vi "Deployment on cDAQ.vi"() -> ()   [LabVIEW 2018]
uses:
  <vilib>/Utility/error.llb/DialogType.ctl
  <vilib>/addons/AML/Data/Common/Controls/aml_Load Data Mode.ctl
  <vilib>/DAQmx/read.llb/DAQmx Read (Analog 2D DBL NChan NSamp).vi
  <vilib>/DAQmx/create/channels.llb/DAQmx Create Channel (AI-Voltage-Basic).vi
  <vilib>/DAQmx/configure/timing.llb/DAQmx Timing (Sample Clock).vi
  <vilib>/DAQmx/miscellaneous.llb/DAQmx Fill In Error Info.vi
  <vilib>/addons/AML/Data/Load Testing Data (2D Array).vi
  <vilib>/addons/AML/Analytics and Machine Learning.lvlib
panel:
  out "Fan status":bool
  out "Predicted probability":dbl[][](array[numeric])=[[0.8062356533229831, 0.19376434667701692]]
  out "Fan status":string="Fan work normal"
  in  "Model file (JSON)":path
  out "Waveform Graph":dbl[][](graph)=[[2.468674629981, 2.468664258944, 2.4700015126559998, 2.469919154421, 2.4675917717059996, 2.4693054330549997, 2.4665564981889996, 2.468985761091, 2.4669664591809997, 2.4659696195069998, 2.466726705208, 2.468710013519, 2.4686398565039998, 2.4688588684029997, 2.468429385459, 2.4684312156419996, 2.467338596391, 2.4671134838819997, 2.4691803705499997, 2.4681774302659996, 2.4676314256709997, 2.46913766628, 2.4677333058579998, 2.467753437871, 2.467754047932, 2.469128515365, 2.4683372662479997, 2.4666229948379996, 2.4670555280869997, 2.466956088144, 2.4668102835649997, 2.46747219975, 2.467281860718, 2.467965129038, 2.4683140839299997, 2.467987701295, 2.4682646689889998, 2.4681414366669996, 2.4681048330069997, 2.4682664991719996, 2.4674844009699997, 2.467387401271, 2.466543686908, 2.4687704095579996, 2.467920594585, 2.4683110336249996, 2.4692737098829998, 2.4674313256629996, 2.4676899915269996, 2.468581290648, 2.468986981213, 2.4680908016039997, 2.468536756195, 2.46729528206, 2.4681987824009997, 2.469066899204, 2.4670829808319996, 2.467718664394, 2.468424504971, 2.466507693309, 2.4675515076799996, 2.4678778903149996, 2.467432545785, 2.4689003525509996, 2.46714276681, 2.4704669891989997, 2.467785161043, 2.467329445476, 2.4664521777579997, 2.467879720498, 2.4686056930879996, 2.467245257058, 2.467746117139, 2.466164839027, 2.466548567396, 2.4686416866869996, 2.4693151940309996, 2.4675655390829996, 2.4688948620019997, 2.468276870209, 2.4672251250449997, 2.467679010429, 2.4681261851419998, 2.4684123037509997, 2.4667260951469996, 2.4670109936339997, 2.467723544882, 2.4679309656219997, 2.469013823897, 2.468553227842, 2.467973059831, 2.4683769202129997, 2.4678004125679998, 2.4687527177889996, 2.46825917844, 2.466208763419, 2.4666534978879997, 2.46754540707, 2.4651307856319997, 2.4662520777499997, 2.4686447369919997, 2.4679077833039997, 2.467624104939, 2.467383740905, 2.4684977122909997, 2.4674923317629998, 2.468615454064, 2.467420344565, 2.4676454570739996, 2.468592881807, 2.467767469274, 2.4686313156499997, 2.4671098235159996, 2.468706353153, 2.466384460987, 2.4665906616049997, 2.4676326457929996, 2.4678644689729996, 2.4684714796679996, 2.469505533063, 2.4686453470529997, 2.4680956820919997, 2.469220024515, 2.466638246363, 2.465340036555, 2.4668993524709997, 2.4679407265979996, 2.4670158741219996, 2.466932295765, 2.469228565369, 2.468526995219, 2.4682427067929997, 2.4690607985939996, 2.4673550680379996, 2.4683226247839998, 2.467491111641, 2.4700741099149996, 2.4665772402629997, 2.4685373662559997, 2.4696013126399996, 2.4668956921049996, 2.4694225647669996, 2.4670018427189997, 2.467727815309, 2.469696482156, 2.4686398565039998, 2.46882043456, 2.4677064631739998, 2.4681542479479996, 2.4683226247839998, 2.469454898, 2.4685648190009997, 2.468633145833, 2.469276150127, 2.4665339259319996, 2.469076050119, 2.4679895314779996, 2.468187801303, 2.467857758302, 2.4675210046299996, 2.4665266052, 2.4667163341709997, 2.467401432674, 2.469397552266, 2.4708104535419997, 2.468003562881, 2.467053697904, 2.4679163241579998, 2.4678327458009996, 2.467182420775, 2.467674129941, 2.4681682793509996, 2.4676460671349996, 2.467580180547, 2.4673141939509997, 2.4672074332759997, 2.4662154740899997, 2.46824087661, 2.46775892842, 2.467804072934, 2.466579070446, 2.4671769302259996, 2.4685373662559997, 2.4678406765939997, 2.4674215646869997, 2.468262838806, 2.46933898641, 2.4683366561869997, 2.4680328458089997, 2.468821654682, 2.467670469575, 2.467735746102, 2.4675771302419998, 2.467866909217, 2.468530655585, 2.4691041129249998, 2.466959138449, 2.465744506998, 2.4680340659309996, 2.4663332158629996, 2.4670512576599997, 2.468821654682, 2.4684763601559996, 2.467526495179, 2.4669664591809997, 2.468500762596, 2.4682567381959997, 2.4678364061669997, 2.46869232175, 2.468008443369, 2.467799802507, 2.467536256155, 2.466900572593, 2.4686575482729998, 2.4677619787249996, 2.4685861711359998, 2.46922307482, 2.4684794104609997, 2.4683189644179997, 2.4686593784559996, 2.469335326044, 2.467544797009, 2.469141936707, 2.4665284353829997, 2.46654490703, 2.4683281153329997, 2.4683451970409998, 2.4668718997259997, 2.4676814506729996, 2.467347137245, 2.469415244035, 2.4674044829789996, 2.4674404765779996, 2.467222684801, 2.467405703101, 2.4669255850939997, 2.4687826107779998, 2.4695512876379997, 2.46870452297, 2.468097512275, 2.468817994316, 2.4665546680059998, 2.467888871413, 2.466838346371, 2.4685379763169997, 2.4702845809599996, 2.468910113527, 2.46742949548, 2.4676491174399997, 2.466312473789, 2.4673690994409996, 2.467219024435, 2.468499542474, 2.467759538481, 2.466347247266, 2.4693109236039996, 2.468580680587, 2.470282140716, 2.467641796708, 2.4675344259719996, 2.4681896314859997, 2.46796024855, 2.468700862604, 2.46645949849, 2.46717937047, 2.466951817717, 2.468650837602, 2.4664485173919997, 2.46703905644, 2.4685062531449997, 2.4680602985539997, 2.468128625386, 2.46827748027, 2.4672110936419998, 2.4677479473219996, 2.4689034028559997, 2.4675478473139996, 2.4668316356999997, 2.4671586283959996, 2.4680419967239997, 2.4678461671429996, 2.4663728698279996, 2.4674667092009996, 2.46878993151, 2.467923034829, 2.467982820807, 2.467722934821, 2.468803962913, 2.466572359775, 2.4670823707709997, 2.466848107347, 2.4680151540399997, 2.4682750400259996, 2.46790534306, 2.4669225347889996, 2.4686099635149996, 2.468469649485, 2.467267219254, 2.46822867539, 2.4693139739089998, 2.467960858611, 2.468397052226, 2.4667425667939997, 2.465985481093, 2.468362278749, 2.46840559308, 2.4666620387419997, 2.4678766701929997, 2.4676088534139997, 2.4677845509819996, 2.467825425069, 2.465226565209, 2.467834575984, 2.468723434861, 2.467732695797, 2.4678284753739996, 2.467093351869, 2.467874229949, 2.468218304353, 2.465888481394, 2.46889364188, 2.468356178139, 2.466468039344, 2.4688100635229997, 2.4681219147149998, 2.466826755212, 2.469374980009, 2.4666309256309997, 2.469415854096, 2.4679718397089996, 2.4679077833039997, 2.4676082433529998, 2.4681505875819996, 2.4664936619059996, 2.467223294862, 2.467782110738, 2.4676271552439997, 2.4679761101359996, 2.468142046728, 2.46895464798, 2.4646488374419997, 2.466418624403, 2.4670915216859997, 2.4681890214249997, 2.4689174342589997, 2.468541026622, 2.4678333558619996, 2.468445857106, 2.467177540287, 2.468018204345, 2.4700747199759996, 2.469173659879, 2.467306873219, 2.4664393664769997, 2.4673904515759997, 2.469022364751, 2.4683598385049996, 2.4669304655819997, 2.466701692707, 2.466473529893, 2.4686325357719996, 2.4675203945689996, 2.466757818319, 2.4668054030769997, 2.4674447470049996, 2.4668908116169996, 2.465874449991, 2.468964408956, 2.4678193244589997, 2.468339706492, 2.468848497366, 2.468179260449, 2.467195232056, 2.468688661384, 2.4677516076879997, 2.466896912227, 2.468722214739, 2.467174489982, 2.46784433696, 2.4665949320319998, 2.4683061531369996, 2.465789651512, 2.469420734584, 2.4686813406519996, 2.469490891599, 2.467505143044, 2.4677174442719996, 2.4667614786849996, 2.468209763499, 2.4673898415149997, 2.466396662207, 2.466651667705, 2.467514293959, 2.468465379058, 2.467329445476, 2.4679077833039997, 2.468384851006, 2.4688015226689997, 2.4679212046459997, 2.467968179343, 2.4661709396369997, 2.468848497366, 2.466919484484, 2.467999292454, 2.4684940519249996, 2.467723544882, 2.4693938919, 2.469108383352, 2.467286741206, 2.4672129238249996, 2.4676979223199997, 2.467373979929, 2.4684306055809997, 2.468620334552, 2.467579570486, 2.4676100735359996, 2.468932075723, 2.4666754600839997, 2.468066399164, 2.468103612885, 2.468022474772, 2.468650837602, 2.4690235848729998, 2.4677198845159998, 2.4665595484939997, 2.467576520181, 2.4692212446369997, 2.468803352852, 2.4676887714049998, 2.467373979929, 2.4679535378789996, 2.4680908016039997, 2.4675643189609997, 2.468848497366, 2.4695744699559996, 2.4676857210999996, 2.4679809906239996, 2.468494661986, 2.4679883113559997, 2.467134836017, 2.4684934418639997, 2.468397662287, 2.468129845508, 2.468709403458, 2.467513073837, 2.4674618287129997, 2.468856428159, 2.467633865915, 2.467080540588, 2.466902402776, 2.467954758001, 2.4683226247839998, 2.4680743299569996, 2.4674630488349996, 2.467942556781, 2.4671628988229997, 2.467275760108, 2.468049317456, 2.4678900915349997, 2.46717937047, 2.4672037729099996, 2.4671275152849996, 2.4685922717459996, 2.468686831201, 2.468929635479, 2.46867401992, 2.4671134838819997, 2.4668322457609997, 2.4672342759599997, 2.467025635098, 2.467054307965, 2.466552837823, 2.4672025527879997, 2.46797244977, 2.466344196961, 2.467450847615, 2.469697092217, 2.468379970518, 2.468848497366, 2.4685916616849997, 2.4677967522019997, 2.466080040548, 2.4669798805229997, 2.4676265451829997, 2.4682744299649997, 2.467677790307, 2.468414133934, 2.465789651512, 2.4693109236039996, 2.465164338987, 2.466901182654, 2.4671043329669997, 2.468682560774, 2.466897522288, 2.468076770201, 2.4662081533579996, 2.4676131238409997, 2.466651667705, 2.467111043638, 2.466536366176], [2.510305044964, 2.5086028436439998, 2.507801161732, 2.5099682653479998, 2.5097754712199998, 2.5073264977079996, 2.51034287166, 2.5084436054559998, 2.5074174038, 2.508483262476, 2.509654669836, 2.5075375950759997, 2.5049165711079997, 2.508780385072, 2.507547966912, 2.5077328296359997, 2.5068402416319997, 2.50811292692, 2.5080262915839997, 2.5092568794199996, 2.50903113946, 2.507720017368, 2.5083337860159998, 2.508718154056, 2.5083783238999997, 2.507791400004, 2.5101049295399998, 2.508482652368, 2.5065577616279997, 2.510592405832, 2.508266674136, 2.5081226886479997, 2.5085040061479997, 2.5069415195599998, 2.5080689991439997, 2.5097345939839997, 2.5089005763479997, 2.5077371003919997, 2.5088895944039997, 2.508569897812, 2.5083478185, 2.5089390131519997, 2.508794417556, 2.508846276736, 2.509361817996, 2.5072056963239997, 2.5068024149359998, 2.5092782332, 2.5086473815279997, 2.50747536406, 2.5084521469679997, 2.507887797068, 2.509170854192, 2.5082459304639997, 2.5079683313239998, 2.5082502012199996, 2.5091452296559997, 2.5094209984719997, 2.50756382972, 2.509106182744, 2.508882273108, 2.510038427768, 2.508191630852, 2.5083221939639997, 2.507802992056, 2.5076852412119996, 2.50790243966, 2.50875354032, 2.5094301500919998, 2.508403948436, 2.5087755042079998, 2.508097064112, 2.509887731092, 2.509689445992, 2.5102684384839997, 2.5065467796839997, 2.5077706563319997, 2.510073814032, 2.507883526312, 2.510220239952, 2.508479601828, 2.5098242798599997, 2.508744998808, 2.5086833778999997, 2.509507633808, 2.508776724424, 2.508175768044, 2.508862139544, 2.508364291416, 2.5088664103, 2.50948872046, 2.507669378404, 2.50861321548, 2.5086113851559997, 2.508544883384, 2.5099902292359997, 2.5089701286599997, 2.507003140468, 2.5094637060319998, 2.509219662832, 2.507274638528, 2.5076968332639997, 2.5097614387359997, 2.510079305004, 2.50860101332, 2.5085393924119996, 2.508486313016, 2.508395406924, 2.5086675150919997, 2.508917659372, 2.5087413381599997, 2.5085064465799998, 2.508865800192, 2.508926810992, 2.508388085628, 2.5095265471559998, 2.509047002268, 2.5072368118319996, 2.5085979627799997, 2.508205053228, 2.510134214724, 2.509145839764, 2.5076992736959998, 2.510655246956, 2.510404492568, 2.5093715797239997, 2.5080122591, 2.511350770076, 2.507895728472, 2.507860952316, 2.506875017788, 2.50744180812, 2.5094277096599997, 2.5095070237, 2.5088920348359998, 2.507917082252, 2.509126316308, 2.508665684768, 2.508484482692, 2.5075851835, 2.508599793104, 2.507144075416, 2.508749269564, 2.506715169492, 2.5082306777639998, 2.508045204932, 2.507047068244, 2.5093697494, 2.5078603422079997, 2.5072685374479997, 2.508181869124, 2.508778554748, 2.5084612985879997, 2.5079164721439997, 2.508929251424, 2.50677373986, 2.509745575928, 2.508184309556, 2.508065948604, 2.508141601996, 2.510163499908, 2.5083893058439997, 2.5101403158039997, 2.509269691688, 2.506792653208, 2.507937215816, 2.5086565331479997, 2.508011038884, 2.508392966492, 2.5104569618559998, 2.5084100495159998, 2.50885725868, 2.508459468264, 2.51003476712, 2.508734016864, 2.5088359048999997, 2.508832244252, 2.509004904816, 2.508098894436, 2.507550407344, 2.5071745808159998, 2.508715713624, 2.5107034454879997, 2.508688868872, 2.5083423275279997, 2.5084655693439997, 2.507934775384, 2.506744454676, 2.5076943928319997, 2.508574168568, 2.507265486908, 2.507533934428, 2.508180648908, 2.508023241044, 2.50832341418, 2.5055309498639997, 2.50763704268, 2.509935929624, 2.509895662496, 2.5090573741039996, 2.509117164688, 2.509039070864, 2.507732219528, 2.50832951526, 2.508774283992, 2.507092216236, 2.507337479652, 2.50892132002, 2.5087572009679997, 2.5089701286599997, 2.507877425232, 2.509428929876, 2.508996363304, 2.507226439996, 2.508578439324, 2.5079542988399997, 2.506448552296, 2.509478348624, 2.5084612985879997, 2.507476584276, 2.508190410636, 2.506696256144, 2.507901829552, 2.508453977292, 2.5099633844839997, 2.508430793188, 2.508605284076, 2.508673616172, 2.509120825336, 2.508938403044, 2.5085400025199998, 2.50884200598, 2.50915926214, 2.509435030956, 2.508897525808, 2.508331955692, 2.50874743924, 2.507744421688, 2.5083783238999997, 2.508616876128, 2.507137974336, 2.5101933952, 2.5082660640279997, 2.508923760452, 2.508151363724, 2.508043374608, 2.509441742144, 2.509154991384, 2.508759031292, 2.5086272479639997, 2.509461875708, 2.5090598145359997, 2.507378966996, 2.508835294792, 2.5086632443359997, 2.50930568806, 2.5103398211199996, 2.506994598956, 2.5093239913, 2.5085003455, 2.509236135748, 2.5087931973399997, 2.507944537112, 2.508488753448, 2.5095399695319998, 2.5088780023519996, 2.5073557828919997, 2.5084295729719996, 2.508212984632, 2.509593048928, 2.508538172196, 2.508139161564, 2.5077236780159997, 2.507806042596, 2.507751132876, 2.5067731297519997, 2.5093605977799998, 2.508324024288, 2.507803602164, 2.508112316812, 2.5074930571919998, 2.51060826864, 2.50745401028, 2.507342970624, 2.509122045552, 2.50919281808, 2.507765775468, 2.50778041806, 2.509926167896, 2.5082416597079997, 2.509967045132, 2.508693749736, 2.508269114568, 2.507828006484, 2.508683988008, 2.5080555767679997, 2.507239862372, 2.511139672708, 2.5080622879559997, 2.5104343878599997, 2.509237966072, 2.5084320134039997, 2.5103806983559998, 2.509143399332, 2.5067865521279997, 2.509460045384, 2.5093355833519997, 2.5087193742719998, 2.507186782976, 2.509804756404, 2.5097144604199997, 2.50918366646, 2.5081745478279998, 2.50874743924, 2.5073533424599996, 2.50812207854, 2.509285554496, 2.5089951430879998, 2.50910740296, 2.508525359928, 2.5065486100079997, 2.5098151282399996, 2.508713273192, 2.5086229772079998, 2.5088334644679997, 2.5087010710319997, 2.50614837916, 2.508026901692, 2.50793294506, 2.509283724172, 2.5064320793799997, 2.5079744324039996, 2.508886543864, 2.5094209984719997, 2.509228814452, 2.508486923124, 2.509301417304, 2.50928128374, 2.508882273108, 2.509222713372, 2.5095149551039997, 2.508847496952, 2.50875354032, 2.5068805087599997, 2.5079902952119997, 2.508208713876, 2.508964637688, 2.508404558544, 2.5094838395959997, 2.508005547912, 2.5076785300239997, 2.50800920856, 2.510164720124, 2.509133027496, 2.5076181293319997, 2.507948807868, 2.508355139796, 2.5091787855959997, 2.5094502836559998, 2.5109182035039996, 2.5088737315959997, 2.5088206522, 2.50759738566, 2.5111225896839997, 2.508859699112, 2.508536341872, 2.508818211768, 2.5079323349519997, 2.5091812260279998, 2.50832951526, 2.5084301830799998, 2.5087931973399997, 2.507985414348, 2.508962197256, 2.5094344208479997, 2.5076919523999996, 2.5076474145159997, 2.508435674052, 2.510002431396, 2.510087236408, 2.508495464636, 2.5095082439159997, 2.5073197865199996, 2.508682157684, 2.5084295729719996, 2.508804789392, 2.5100561209, 2.509652229404, 2.5098273304, 2.508910338076, 2.5086296883959998, 2.5090195474079997, 2.508119638108, 2.5078243458359997, 2.508297179536, 2.506585826596, 2.507511360432, 2.5087102226519997, 2.509447233116, 2.5083356163399997, 2.509976196752, 2.508834074576, 2.5084588581559997, 2.50692626686, 2.5083716127119997, 2.509796214892, 2.50857050792, 2.508292298672, 2.511378835044, 2.510619860692, 2.5089951430879998, 2.5074997683799998, 2.50742045434, 2.50915316106, 2.510860853352, 2.509144619548, 2.5092306447759998, 2.5093020274119997, 2.5083423275279997, 2.5065479999, 2.5078652230719998, 2.5075083098919997, 2.5071611584399998, 2.507173970708, 2.5081922409599997, 2.5083270748279998, 2.5069817866879998, 2.507282569932, 2.508192851068, 2.5092214931559997, 2.508759031292, 2.507497938056, 2.507918302468, 2.506427198516, 2.508522919496, 2.509260540068, 2.508751709996, 2.50814648286, 2.508453367184, 2.5073155157639997, 2.5084344538359997, 2.509600980332, 2.508874341704, 2.507766995684, 2.509352056268, 2.509899323144, 2.506900032216, 2.509984128156, 2.50882370274, 2.5094948215399997, 2.5091470599799996, 2.508303890724, 2.50831426256, 2.508839565548, 2.509029309136, 2.5105289546, 2.5099231173559997, 2.507686461428, 2.5091318072799997, 2.5090012441679996, 2.508334396124, 2.5107571349919997, 2.509036020324, 2.5084612985879997, 2.507639483112, 2.507917082252, 2.50854305306, 2.509128146632, 2.507676089592, 2.5090061250319997, 2.509480789056, 2.509148890304, 2.510137265264, 2.5083478185, 2.509910305088, 2.5088108904719997, 2.5076089777119996, 2.50613312646, 2.5081605153439996, 2.5067157796, 2.507137974336, 2.509011616004, 2.509446623008, 2.507798111192, 2.5092031899159997, 2.509440521928, 2.5081470929679996, 2.5092642007159998, 2.508108046056, 2.51020254682, 2.50911960512, 2.5077346599599997, 2.5059970723759997, 2.509532038128, 2.5087260854599998, 2.5091543812759998, 2.5085393924119996, 2.508881052892, 2.506881118868, 2.509491771]]
  in  "Stop":bool
  in  "Number of Samples":i32=500
  in  "Sample Rate":dbl=1000.0
  in  "Sample Clock Source":tag="OnboardClock"
  in  "Physical Channel":tag="cDAQ9188-18973A7Mod2/ai0:1"
  # "Fan Fault Detection: Deployment"
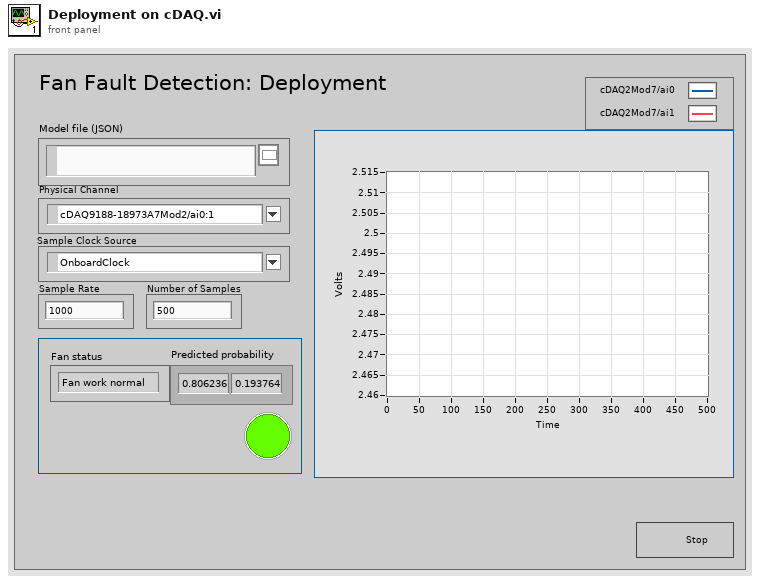
[diagram p1: front panel]
types:
  T1 = typedef "DialogType.ctl" = u16
  T2 = typedef "Analytics and Machine Learning.lvlib/aml_Load Data Mode.ctl" = u16
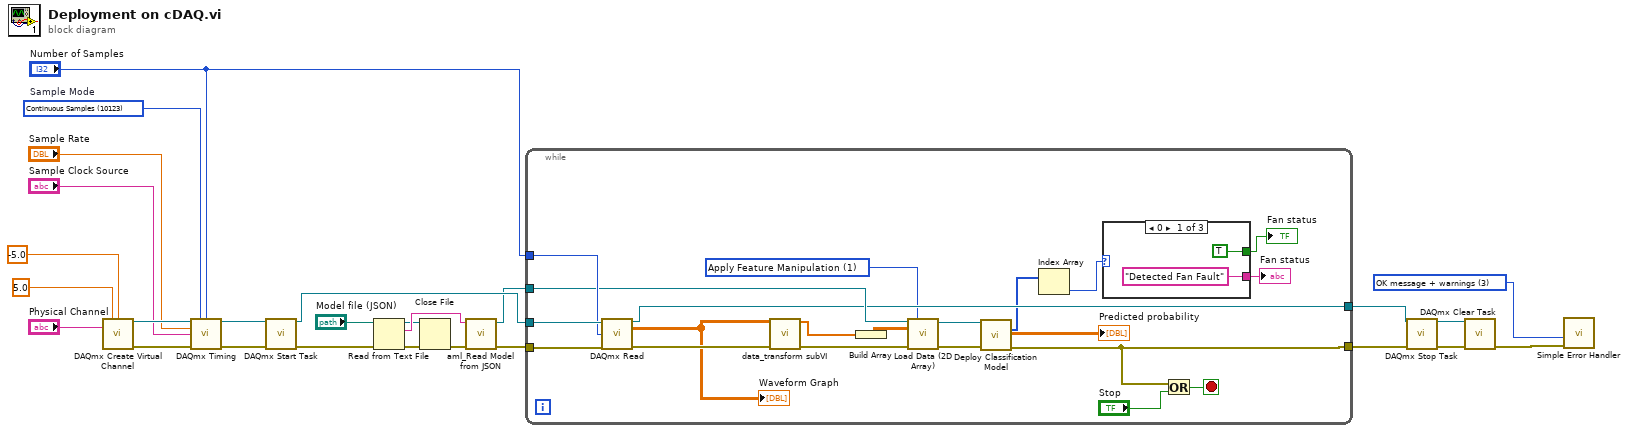
[diagram p0: block diagram]
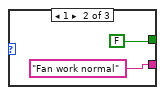
[diagram p2: hidden frame]
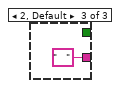
[diagram p3: hidden frame]
diagram:
  w14 = T1 3 items=["no dialog", "OK message", "continue or stop message", "OK message + warnings", "continue/stop + warnings"] ("type of dialog (OK msg:1)")
  w26 = 10123 items=["Finite Samples"=10178, "Continuous Samples"=10123, "Hardware Timed Single Point"=12522]  # Sample Mode
  n1 = call-poly <vilib>:"DAQmx Create Virtual Channel.vi"("maximum value"=5.0 ("Max Voltage"), "minimum value"=-5.0 ("Min Voltage"), "physical channels"="Physical Channel") -> ("task out"=w24:refnum<k21>, "error out"=w25:errorcluster)  [unwired: 11 in]
  n2 = call-poly <vilib>:"DAQmx Timing.vi"("task/channels in"=w24, "sample mode"=w26, "samples per channel"="Number of Samples", "rate"="Sample Rate", "source"="Sample Clock Source", "error in"=w25) -> ("task out"=w13:refnum<k21>, "error out"=w12:errorcluster)  [unwired: 8 in]
  n3 = call <vilib>:"DAQmx Start Task.vi"("task/channels in"=w13, "error in"=w12) -> ("task out"=w10:refnum<k21>, "error out"=w9:errorcluster)  [unwired: 12 in]
  n4 = Read from Text File(file (use dialog)="Model file (JSON)", error in=w9) -> (refnum out=w3:refnum<file>, text=w4:string, error out=w2:errorcluster)  [unwired: 2 in, 1 out]
  n5 = Close File(refnum=w3, error in=w2) -> (error out=w5:errorcluster)  [unwired: 1 out]
  n6 = call <vilib>:"aml_Read Model from JSON.vi"("error in (no error)"=w5, "JSON string"=w4) -> ("error out"=w11:errorcluster, "model out"=w8:refnum<class "AML Analytics Model.lvclass">)  [unwired: 6 in, 2 out]
  n7 = while {
    tunnel: w10 -> [w47]
    tunnel: w11 -> [w46]
    tunnel: "Number of Samples" -> [w43]
    tunnel: w8 -> [w42]
    tunnel: [w41] -> w7
    tunnel: [w33] -> w6
    stop <- w44 stop-if-true
    w34 = T2 1 items=["Read Raw Data", "Apply Feature Manipulation"] ("load data mode")
    n8 = call-poly <vilib>:"DAQmx Read.vi"("task/channels in"=w47, "number of samples per channel"=w43, "error in"=w46) -> ("task out"=w41:refnum<k21>, "data"=w27:dbl[][], "error out"=w30:errorcluster)  [unwired: 10 in]
    "Waveform Graph" <- w27
    n9 = call "data_transform subVI.vi"("data"=w27, "error in (no error)"=w30) -> ("Array"=w28:dbl[], "error out"=w29:errorcluster)  [unwired: 12 in]
    n10 = Build Array(w28) -> (w38:dbl[][])
    n11 = call-poly <vilib>:"Load Data (2D Array).vi"("model in"=w42, "load data mode"=w34, "data"=w38, "error in (no error)"=w29) -> ("model out"=w40:refnum<class "AML Analytics Model.lvclass">, "error out"=w39:errorcluster)  [unwired: 10 in]
    n12 = call <vilib>:"Deploy Classification Model.vi"("model in"=w40, "error in (no error)"=w39) -> ("predicted labels"=w37:i32[], "predicted probabilities"=→"Predicted probability":dbl[][], "error out"=w33:errorcluster)  [unwired: 10 in, 1 out]
    n13 = Index Array(array=w37) -> (element=w36:i32)  [unwired: 1 in]
    n14 = case shown="0" w36 {
      tunnel: ["Detected Fan Fault" "Fan work normal" "   "] -> w35
      tunnel: [TRUE FALSE _] -> w31
      frame 0 {
      }
      frame 1 {
      }
      frame 2, Default {
      }
    }
    "Fan status" <- w35
    "Fan status" <- w31
    n15 = Or(x=w33, y="Stop") -> (x .or. y?=w44:bool)
  }
  n16 = call <vilib>:"DAQmx Stop Task.vi"("task/channels in"=w7, "error in"=w6) -> ("task out"=w15:refnum<k21>, "error out"=w16:errorcluster)  [unwired: 12 in]
  n17 = call <vilib>:"DAQmx Clear Task.vi"("task in"=w15, "error in"=w16) -> ("error out"=w23:errorcluster)  [unwired: 13 in]
  n18 = call <vilib>:"Simple Error Handler.vi"("type of dialog (OK msg:1)"=w14, "error in (no error)"=w23) -> ()  [unwired: 3 in, 5 out]
